vi "Create.vi"(8 "error in (no error)":errorcluster, 10 "Msg Q":refnum<class "MessageQ.lvclass">) -> (0 "error out":errorcluster, 3 "SequencingHttpCtrlr out":refnum<class "SequencingHttpCtrlr.lvclass">)   [LabVIEW 2020, in "VolatusSeq.lvlib" / "SequencingHttpCtrlr.lvclass"]
uses:
  SequencingHttpCtrlr.lvclass
  SequencingHttpCtrlr.lvclass/SequencingHttpCtrlr.ctl
  Volatus/MessageQ/MessageQ.lvclass
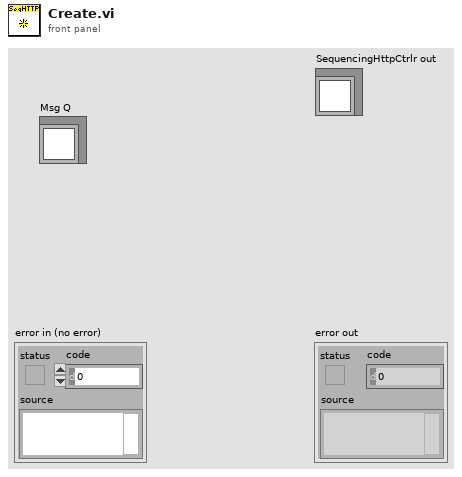
[diagram p1: front panel]
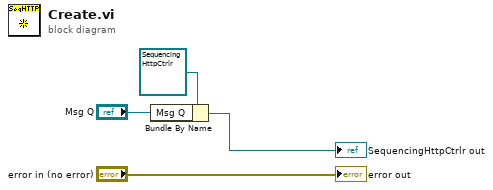
[diagram p0: block diagram]
diagram:
  n1 = Bundle By Name(cluster=refnum<class "SequencingHttpCtrlr.lvclass"> refnum ("SequencingHttpCtrlr in"), "Msg Q"="Msg Q") -> (→"SequencingHttpCtrlr out":refnum<class "SequencingHttpCtrlr.lvclass">)
  "error out" <- "error in (no error)"
